vi "disconnectFromComponent.vi"(8 "error in":errorcluster, 11 "MiddlewareSALThisComponent.lvclass in":refnum<class "MiddlewareSALThisComponent.lvclass">) -> (0 "error out":errorcluster, 3 "MiddlewareSALThisComponent.lvclass out":refnum<class "MiddlewareSALThisComponent.lvclass">)   [LabVIEW 2016, in "MiddlewareSALThisComponent.lvclass"]
uses:
  MiddlewareSALThisComponent.lvclass
  ts_sallv_exa/SALLV_EXA.lvlib
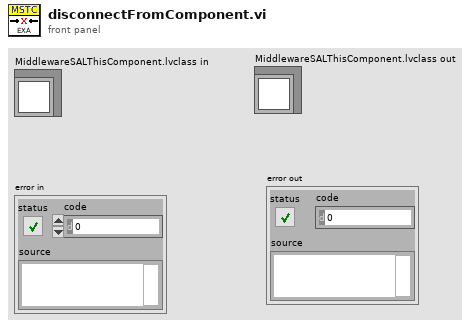
[diagram p1: front panel]
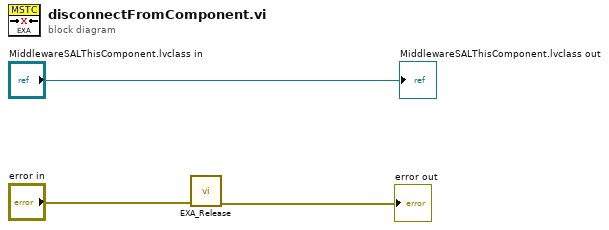
[diagram p0: block diagram]
diagram:
  n1 = call "EXA_Release.vi"("error in (no error)"="error in") -> ("error out"=→"error out":errorcluster)  [unwired: 9 in, 1 out]
  "MiddlewareSALThisComponent.lvclass out" <- "MiddlewareSALThisComponent.lvclass in"
